vi "UpdateTimingPlot.vi"(2 "Ctl Refnum":refnum<vi>, 3 "TimingArray":T1 {"Timing Sequence"."Dt" format="%_3p"; "Timing Sequence"."Time" format="%_3p"}) -> ()   [LabVIEW 2014]
uses:
  Controls/TimingControlArray.ctl
  Controls/TimingControl.ctl
  Controls/TimingControlChannel.ctl
  Controls/TimingPlotData.ctl
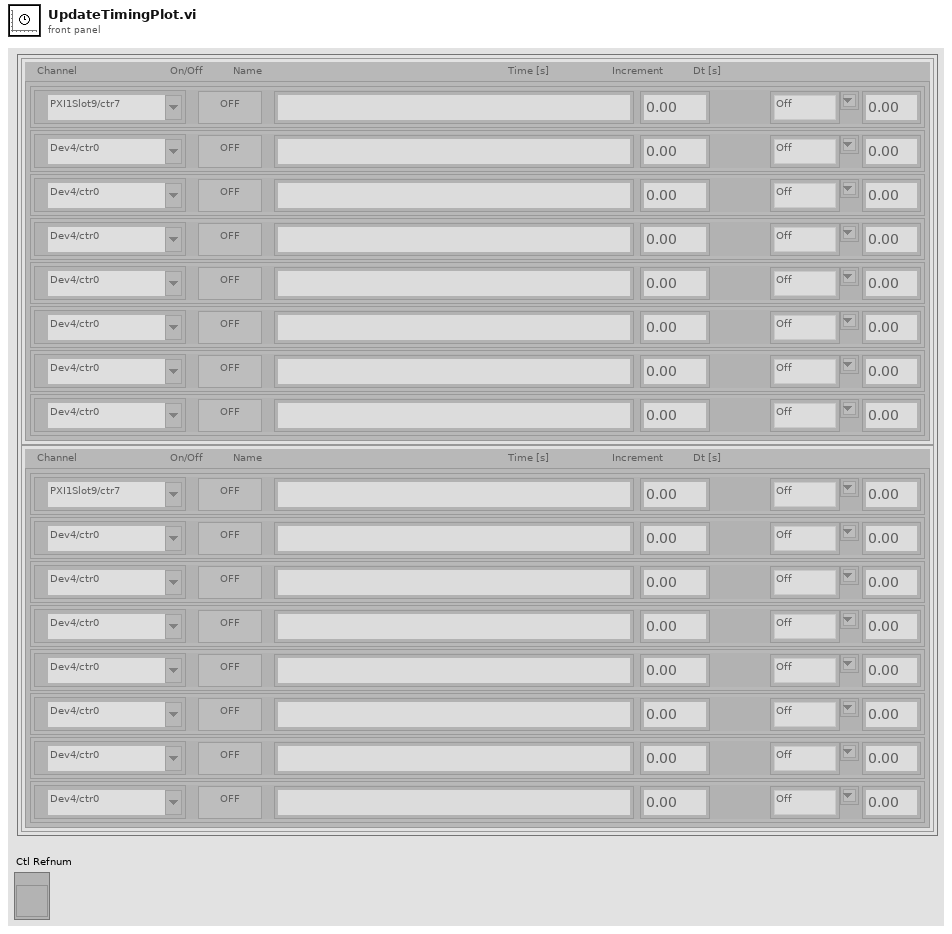
[diagram p1: front panel]
types:
  T1 = typedef "TimingControlArray.ctl" = T2[]
  T2 = typedef "TimingControl.ctl" = cluster{"Timing Sequence":T3[]}
  T3 = typedef "TimingControlChannel.ctl" = cluster{"Active":bool, "counter":tag, "Channel Name":string, "Time":dbl, "Increment":string, "Dt":dbl}
  T4 = typedef "TimingPlotData.ctl" = cluster{"Time":dbl, "Name":string, "Active":bool}
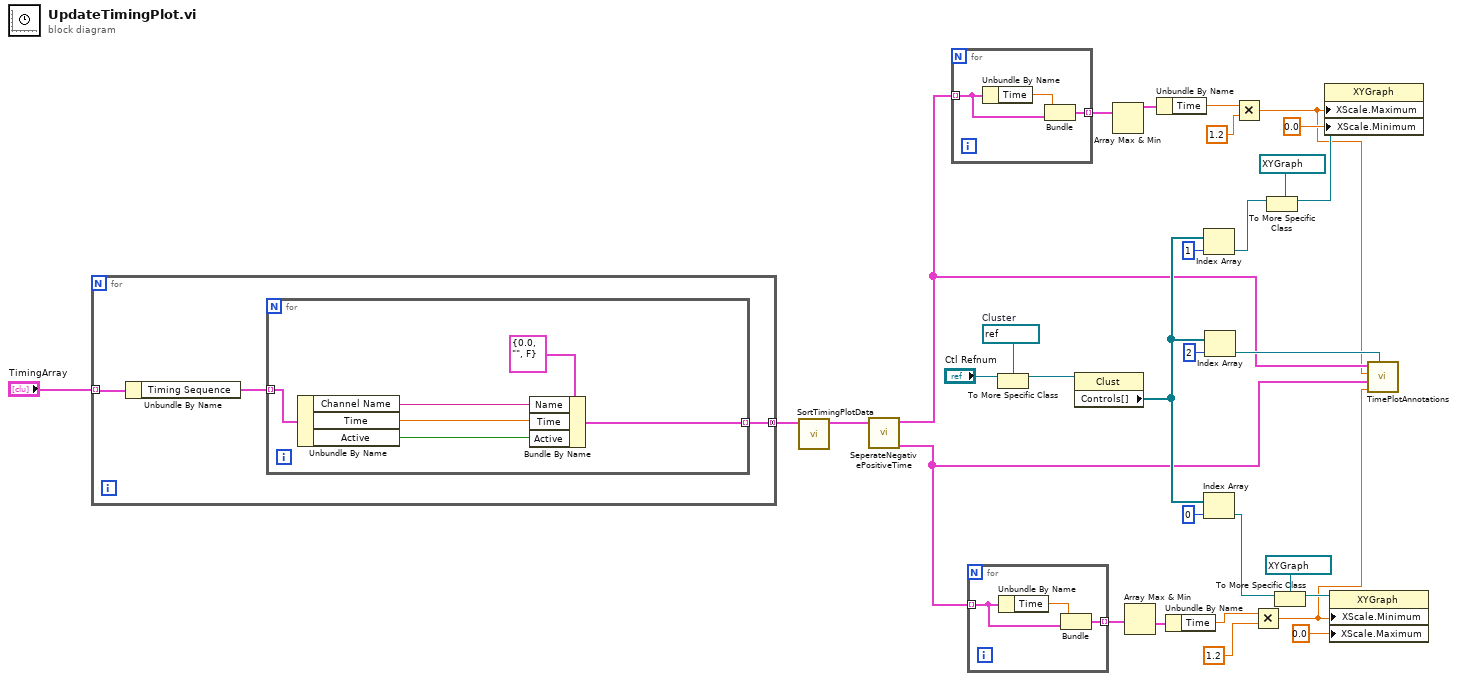
[diagram p0: block diagram]
diagram:
  w2 = refnum<vi> refnum  # Cluster
  n1 = for {
    tunnel: "TimingArray" -> [w34] mode=indexing
    tunnel: [w32] -> w19 mode=concatenating
    n2 = Unbundle By Name(w34) -> ("Timing Sequence"=w33:T3[])
    n3 = for {
      tunnel: w33 -> [w40] mode=indexing
      tunnel: [w36] -> w32 mode=indexing
      n4 = Unbundle By Name(w40) -> ("Channel Name"=w39:string, "Time"=w38:dbl, "Active"=w37:bool)
      n5 = Bundle By Name(cluster=T4 {"Time"=0.0, "Name"="", "Active"=FALSE} ("TimingPlotData"), "Name"=w39, "Time"=w38, "Active"=w37) -> (w36:T4)
    }
  }
  n6 = call "SortTimingPlotData.vi"("TimingPlotData"=w19) -> ("SortedTimingPlotData"=w18:T4[])  [unwired: 10 in]
  n7 = call "SeperateNegativePositiveTime.vi"("TimePlotData"=w18) -> ("Negative TimePlotData"=w6:T4[], "Positive TimePlotData"=w7:T4[])  [unwired: 9 in]
  n8 = for {
    tunnel: w7 -> [w42] mode=indexing
    tunnel: [w41] -> w13 mode=indexing
    n9 = Unbundle By Name(w42) -> ("Time"=w43:dbl)
    n10 = Bundle("Time"=w43, "TimingPlotData"=w42) -> (w41:cluster{"Time":dbl, "TimingPlotData":T4})  [unwired: 1 in]
  }
  n11 = for {
    tunnel: w6 -> [w45] mode=indexing
    tunnel: [w44] -> w17 mode=indexing
    n12 = Unbundle By Name(w45) -> ("Time"=w46:dbl)
    n13 = Bundle("Time"=w46, "TimingPlotData"=w45) -> (w44:cluster{"Time":dbl, "TimingPlotData":T4})  [unwired: 1 in]
  }
  n14 = To More Specific Class(target class=w2, reference="Ctl Refnum") -> (specific class reference=w1:refnum<vi>)  [unwired: 1 in, 1 out]
  n15 = property class="Clust"(reference=w1) -> ("Controls[]"=w10:refnum<vi>[])  [unwired: 1 in, 2 out]
  n16 = Array Max & Min(array=w13) -> (max value=w12:cluster{"Time":dbl, "TimingPlotData":T4})  [unwired: 3 out]
  n17 = Array Max & Min(array=w17) -> (min value=w16:cluster{"Time":dbl, "TimingPlotData":T4})  [unwired: 3 out]
  n18 = Unbundle By Name(w12) -> ("Time"=w11:dbl)
  n19 = Unbundle By Name(w16) -> ("Time"=w15:dbl)
  n20 = Index Array(array=w10, index=1) -> (element=w14:refnum<vi>)
  n21 = Index Array(array=w10, index=0) -> (element=w27:refnum<vi>)
  n22 = Index Array(array=w10, index=2) -> (element=w8:refnum<vi>)
  n23 = Multiply(x=w11, y=1.2) -> (x*y=w4:dbl)
  n24 = Multiply(x=w15, y=1.2) -> (x*y=w5:dbl)
  n25 = To More Specific Class(target class=refnum<vi> refnum, reference=w14) -> (specific class reference=w25:refnum<vi>)  [unwired: 1 in, 1 out]
  n26 = To More Specific Class(target class=refnum<vi> refnum, reference=w27) -> (specific class reference=w29:refnum<vi>)  [unwired: 1 in, 1 out]
  n27 = property class="XYGraph"(reference=w25, "XScale.Maximum"=w4, "XScale.Minimum"=0.0 ("X Scale.Range:Minimum")) -> ()  [unwired: 1 in, 2 out]
  n28 = property class="XYGraph"(reference=w29, "XScale.Minimum"=w5, "XScale.Maximum"=0.0 ("X Scale.Range:Maximum")) -> ()  [unwired: 1 in, 2 out]
  n29 = call "TimePlotAnnotations.vi"("Top Plot"=w8, "Negative Min"=w5, "Negative TimingPlotData"=w6, "Postitive Max"=w4, "Positive TimingPlotData"=w7) -> ()  [unwired: 7 in]
